vi "Translate to Array Data.vi"(0 "original data":path=path "C:/Users/User/Desktop/aaa.csv", 1 "Only Use Last Value?":bool=TRUE, 2 "Electrode number, N":u16=8, 3 "Current Mode":u8[][](array[numeric]), 5 "original error":errorcluster, 7 "Array Mode":u16(ring) items=["None", "Gradient + Dipole dipole", "Gradient", "Dipole Dipole", "Schlumberger"], 9 "modified data":path=path "C:/Users/User/Desktop/test.csv", 11 "modified error":errorcluster, 12 "Inverse\nPolarity":bool=TRUE, 13 "Insert\nBreak":bool=TRUE, 14 "External\nRef":bool=TRUE) -> ()   [LabVIEW 2023]
uses:
  <vilib>/Utility/error.llb/DialogType.ctl
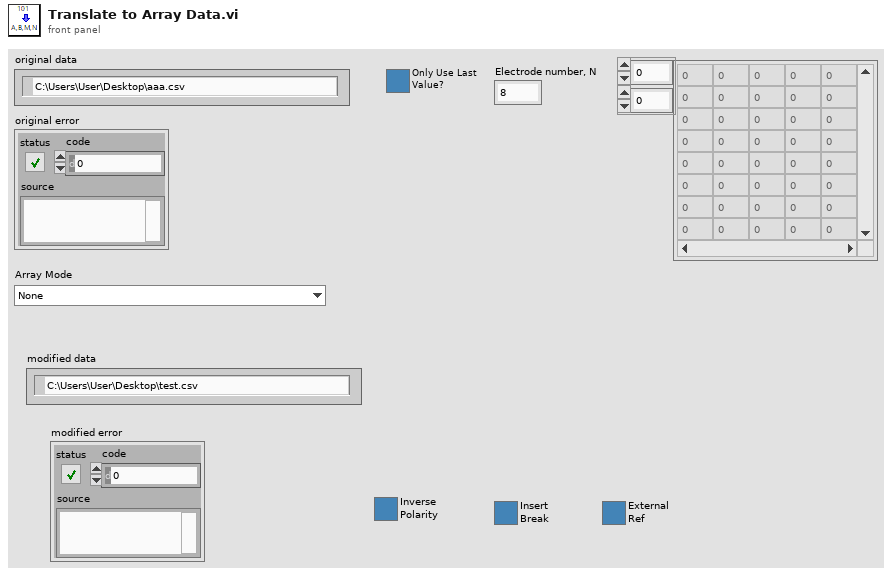
[diagram p1: front panel]
types:
  T1 = enum16{"open", "replace", "create", "open or create", "replace or create", "replace or create with confirmation"}
  T2 = typedef "DialogType.ctl" = u16
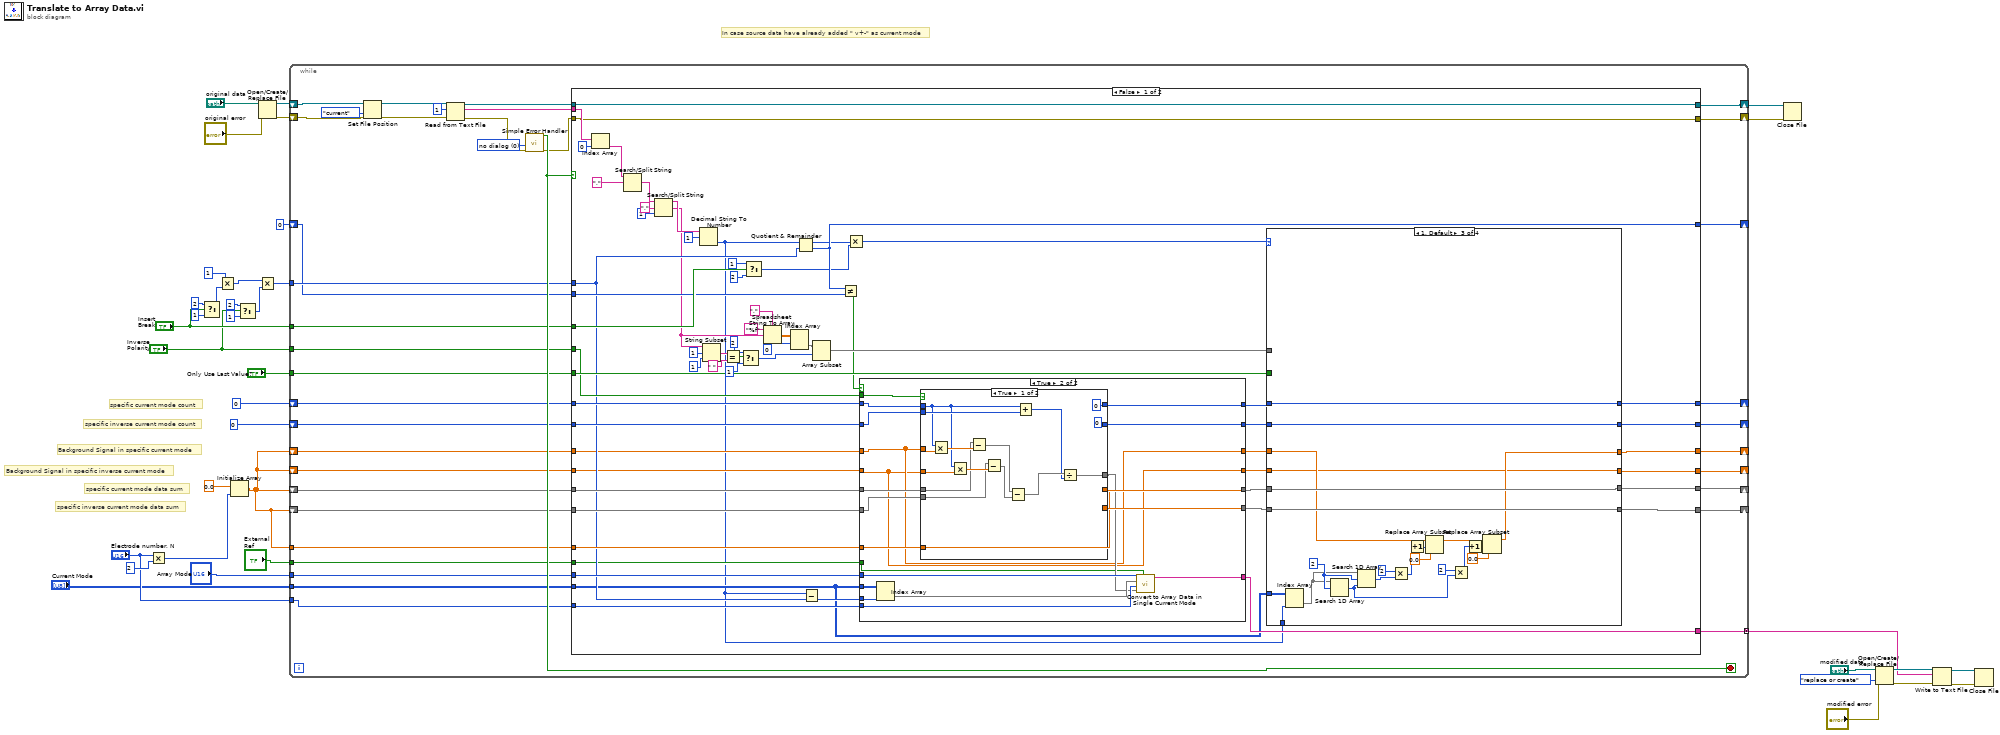
[diagram p0: block diagram]
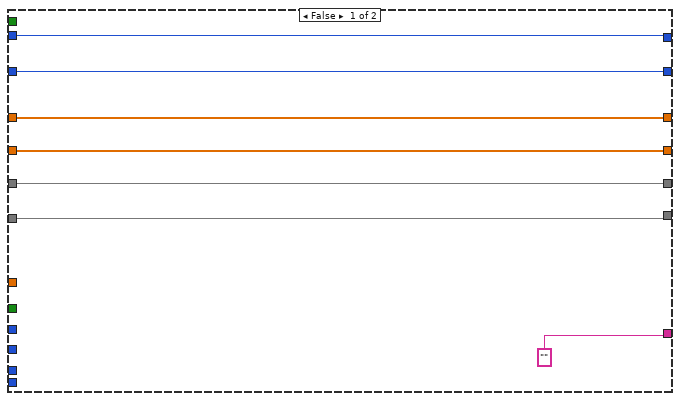
[diagram p2: hidden frame]
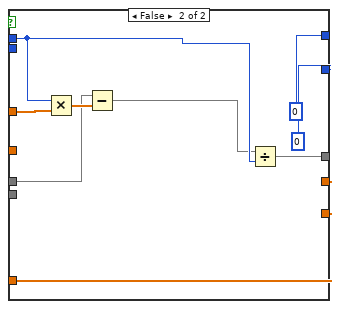
[diagram p3: hidden frame]
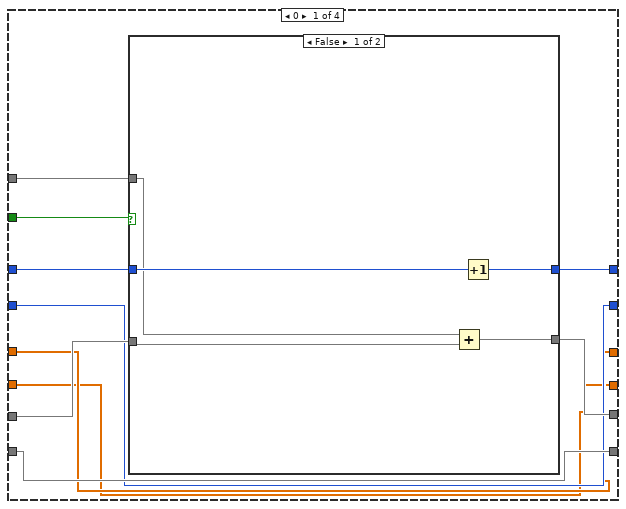
[diagram p4: hidden frame]
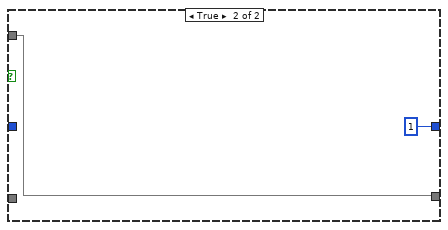
[diagram p5: hidden frame]
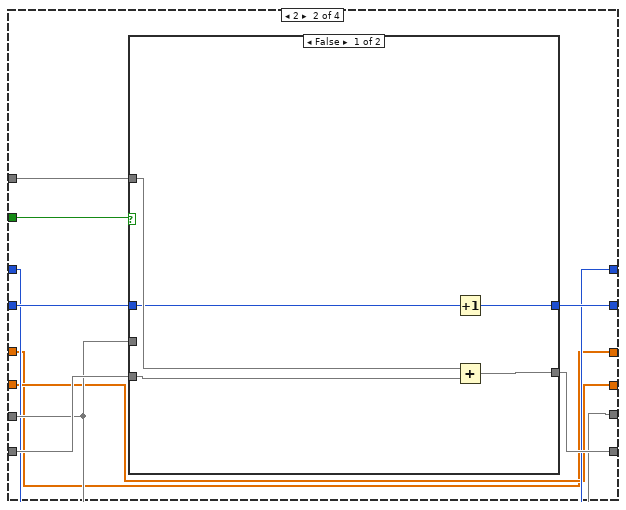
[diagram p6: hidden frame]
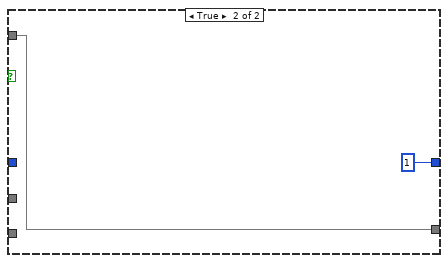
[diagram p7: hidden frame]
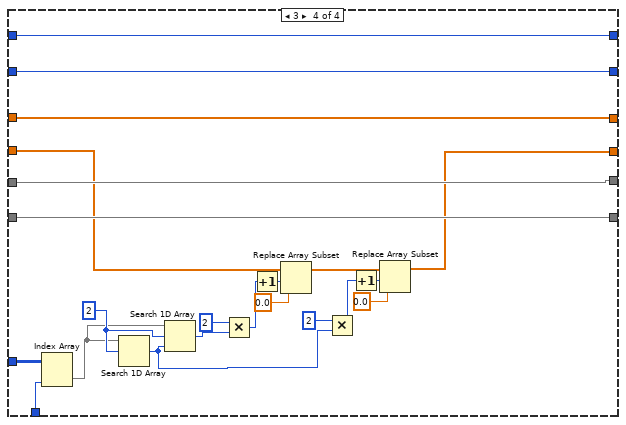
[diagram p8: hidden frame]
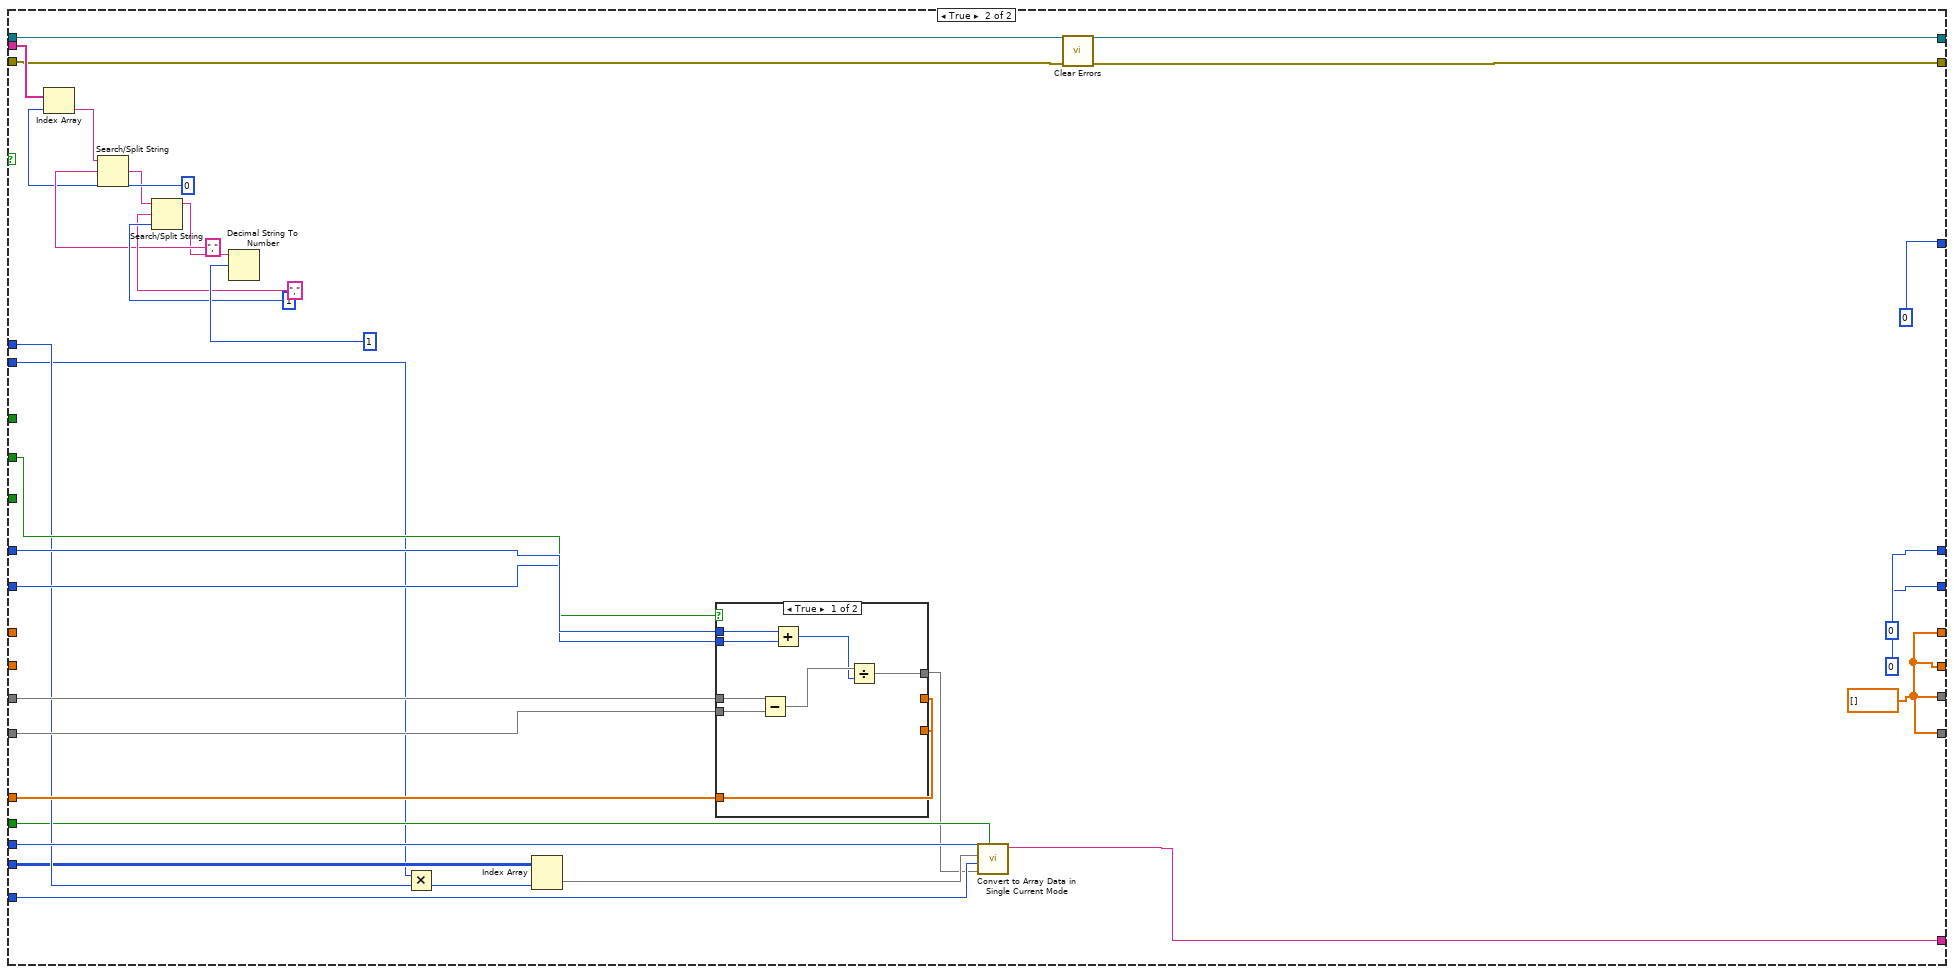
[diagram p9: hidden frame]
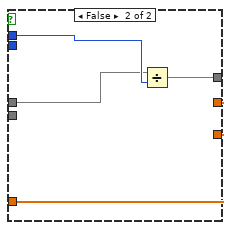
[diagram p10: hidden frame]
diagram:
  # "Background Signal in specific inverse current mode"
  # "Background Signal in specific current mode"
  # "In case source data have already added \" v+-\" as current mode"
  # "specific inverse current mode data sum"
  # "specific current mode data sum"
  # "specific inverse current mode count"
  # "specific current mode count"
  n1 = Multiply(x="Electrode number, N", y=u16 2) -> (x*y=w11:u16)
  n2 = Select(t=2 ("number"), s="Insert\nBreak", f=1 ("number")) -> (s? t:f=w20:i32)
  n3 = Multiply(x=1 ("number"), y=w20) -> (x*y=w14:i32)
  n4 = Initialize Array(0.0 ("element"), w11) -> (w1:dbl[])
  n5 = Select(t=2 ("number"), s="Inverse\nPolarity", f=1 ("number")) -> (s? t:f=w19:i32)
  n6 = Open/Create/Replace File(file path (use dialog)="original data", error in="original error") -> (refnum out=w34:refnum<file>, error out=w35:errorcluster)  [unwired: 4 in, 1 out]
  n7 = Multiply(x=w14, y=w19) -> (x*y=w18:i32)
  n8 = while {
    shift-right: [w67] -> w29
    shift-left: w35 -> [w74]
    shift-right: [w66] -> w36
    shift-left: w34 -> [w65]
    tunnel: "Insert\nBreak" -> [w61]
    tunnel: "Inverse\nPolarity" -> [w60]
    tunnel: "Only Use Last Value?" -> [w59]
    tunnel: w18 -> [w58]
    shift-right: [w53] -> _
    shift-left: 0 ("number") -> [w57]
    shift-right: [w50] -> _
    shift-left: 0 ("number") -> [w56]
    shift-right: [w52] -> _
    shift-left: w1 -> [w55]
    shift-right: [w51] -> _
    shift-left: w1 -> [w54]
    shift-right: [w49] -> _
    shift-left: 0 -> [w48]
    tunnel: w1 -> [w47]
    tunnel: "Current Mode" -> [w45]
    tunnel: "Array Mode" -> [w46]
    tunnel: "Electrode number, N" -> [w44]
    tunnel: "External\nRef" -> [w43]
    tunnel: [w42] -> w5 mode=concatenating
    shift-right: [w39] -> _
    shift-left: w1 -> [w41]
    shift-right: [w38] -> _
    shift-left: w1 -> [w40]
    stop <- w71 stop-if-true
    w72 = T2 0 items=["no dialog", "OK message", "continue or stop message", "OK message + warnings", "continue/stop + warnings"] ("type of dialog (OK msg:1)")
    n9 = Set File Position(refnum=w65, from (0:start)=enum16{"start", "end", "current"}."current", error in=w74) -> (refnum out=w64:refnum<file>, error out=w63:errorcluster)  [unwired: 1 in]
    n10 = Read from Text File(file (use dialog)=w64, count=1, error in=w63) -> (refnum out=w69:refnum<file>, text=w70:string[], error out=w68:errorcluster)  [unwired: 1 in, 1 out]
    n11 = call <vilib>:"Simple Error Handler.vi"("type of dialog (OK msg:1)"=w72, "error in (no error)"=w68) -> ("error?"=w71:bool, "error out"=w62:errorcluster)  [unwired: 3 in, 3 out]
    n12 = case shown="False" w71 {
      tunnel: w70 -> [w135 w297]
      tunnel: w69 -> [w132 w294]
      tunnel: w62 -> [w131 w276]
      tunnel: [w132 w294] -> w66
      tunnel: [w131 w275] -> w67
      tunnel: w61 -> [w128 _]
      tunnel: w60 -> [w108 w287]
      tunnel: w59 -> [w127 _]
      tunnel: w58 -> [w96 w283]
      tunnel: w57 -> [w112 w291]
      tunnel: w56 -> [w111 w290]
      tunnel: w55 -> [w110 w289]
      tunnel: w54 -> [w109 w288]
      tunnel: [w118 0 ("number")] -> w53
      tunnel: [w117 w270] -> w52
      tunnel: [w116 w270] -> w51
      tunnel: [w115 0 ("number")] -> w50
      tunnel: [w113 0] -> w49
      tunnel: w48 -> [w114 w271]
      tunnel: w47 -> [w102 w286]
      tunnel: w46 -> [w98 w285]
      tunnel: w45 -> [w79 w272]
      tunnel: w44 -> [w95 w282]
      tunnel: w43 -> [w94 w281]
      tunnel: [w93 w280] -> w42
      tunnel: w41 -> [w83 _]
      tunnel: w40 -> [w82 _]
      tunnel: [w77 w270] -> w39
      tunnel: [w76 w270] -> w38
      frame False {
        n13 = Index Array(array=w135, index=0) -> (element=w133:string)
        n14 = Search/Split String(string=w133, search string/char (-)=",") -> (match + rest of string=w123:string)  [unwired: 1 in, 2 out]
        n15 = Search/Split String(string=w123, search string/char (-)=",", offset (0)=1) -> (substring before match=w124:string, match + rest of string=w85:string)  [unwired: 1 out]
        n16 = Decimal String To Number(string=w124, offset=1) -> (number=w78:i32)  [unwired: 1 in, 1 out]
        n17 = String Subset(string=w85, offset (0)=1, length (rest)=1 ("length (rest)")) -> (substring=w92:string)
        n18 = Equal?(x=w92, y=" ") -> (x = y?=w91:bool)
        n19 = Select(t=2 ("index (row)"), s=w91, f=1 ("index (row)")) -> (s? t:f=w84:i32)
        n20 = Select(t=1, s=w128, f=2 ("y")) -> (s? t:f=w101:i32)
        n21 = Spreadsheet String To Array(delimiter (Tab)=",", format string="%f", spreadsheet string=w85) -> (array=w122:dbl[][])  [unwired: 1 in]
        n22 = Index Array(array=w122, index (row)=0) -> (element=w120:dbl[])  [unwired: 1 in]
        n23 = Quotient & Remainder(x=w78, y=w96) -> (x-y*floor(x/y)=w100:i32, floor(x/y)=w113:i32)
        n24 = Subtract(x=w78, y=w96) -> (x-y=w97:i32)
        n25 = Array Subset(array=w120, index=w84) -> (w119:dbl[])  [unwired: 1 in]
        n26 = Not Equal?(x=w113, y=w114) -> (x != y?=w103:bool)
        n27 = Multiply(x=w100, y=w101) -> (x*y=w99:i32)
        n28 = case shown="True" w103 {
          tunnel: w112 -> [w146 w163]
          tunnel: w111 -> [w145 w162]
          tunnel: w110 -> [w144 w165]
          tunnel: w109 -> [w143 w164]
          tunnel: w108 -> [_ w166]
          tunnel: [w146 w161] -> w107
          tunnel: [w145 w160] -> w106
          tunnel: [w144 w159] -> w105
          tunnel: [w143 w158] -> w104
          tunnel: w102 -> [_ w157]
          tunnel: w98 -> [_ w153]
          tunnel: w79 -> [_ w156]
          tunnel: w97 -> [_ w155]
          tunnel: w95 -> [_ w152]
          tunnel: w94 -> [_ w150]
          tunnel: ["" ("String") w149] -> w93
          tunnel: w83 -> [w141 w148]
          tunnel: w82 -> [w140 w147]
          tunnel: [w141 w148] -> w81
          tunnel: [w140 w147] -> w80
          frame False {
          }
          frame True {
            n29 = Index Array(array=w156, index (col)=w155) -> (element=w154:u8[])  [unwired: 1 in]
            n30 = case shown="True" w166 {
              tunnel: w165 -> [w170 w184]
              tunnel: w164 -> [w169 _]
              tunnel: w163 -> [w171 w186]
              tunnel: w162 -> [w182 _]
              tunnel: [0 ("number") 0 ("number")] -> w161
              tunnel: [0 ("number") 0 ("number")] -> w160
              tunnel: [w177 w189] -> w159
              tunnel: [w177 w189] -> w158
              tunnel: w157 -> [w177 w189]
              tunnel: [w176 w188] -> w151
              tunnel: w148 -> [w174 w187]
              tunnel: w147 -> [w172 _]
              frame True {
                n31 = Multiply(x=w171, y=w174) -> (x*y=w175:dbl[])
                n32 = Multiply(x=w171, y=w172) -> (x*y=w173:dbl[])
                n33 = Subtract(x=w170, y=w175) -> (x-y=w167:dbl[])
                n34 = Subtract(x=w169, y=w173) -> (x-y=w168:dbl[])
                n35 = Subtract(x=w167, y=w168) -> (x-y=w181:dbl[])
                n36 = Add(x=w171, y=w182) -> (x+y=w180:i32)
                n37 = Divide(x=w181, y=w180) -> (x/y=w176:dbl[])
              }
              frame False {
                n38 = Multiply(x=w186, y=w187) -> (x*y=w185:dbl[])
                n39 = Subtract(x=w184, y=w185) -> (x-y=w183:dbl[])
                n40 = Divide(x=w183, y=w186) -> (x/y=w188:dbl[])
              }
            }
            n41 = call "Convert to Array Data in Single Current Mode.vi"("External\nRef"=w150, "data"=w151, "Electrode number, N"=w152, "Current Mode"=w154, "Array Mode"=w153) -> ("String"=w149:string)  [unwired: 6 in]
          }
        }
        n42 = case shown="1, Default" w99 {
          tunnel: w127 -> [w201 w218 _ _]
          tunnel: w119 -> [w197 w217 _ _]
          tunnel: w107 -> [w200 w211 w247 w269]
          tunnel: w106 -> [w194 w214 w246 w268]
          tunnel: w105 -> [w199 w212 w245 w267]
          tunnel: w104 -> [w195 w216 w244 w266]
          tunnel: [w198 w211 w247 w269] -> w118
          tunnel: [w196 w212 w245 w267] -> w117
          tunnel: [w195 w215 w244 w266] -> w116
          tunnel: [w194 w213 w246 w268] -> w115
          tunnel: w81 -> [w193 w209 w239 w248]
          tunnel: w80 -> [w192 w210 w226 w250]
          tunnel: w79 -> [_ _ w241 w263]
          tunnel: w78 -> [_ _ w240 w262]
          tunnel: [w193 w209 w227 w248] -> w77
          tunnel: [w192 w210 w226 w249] -> w76
          frame 0 {
            n43 = case shown="False" w201 {
              tunnel: w200 -> [w206 _]
              tunnel: w199 -> [w203 _]
              tunnel: [w205 1 ("number")] -> w198
              tunnel: w197 -> [w202 w207]
              tunnel: [w204 w207] -> w196
              frame False {
                n44 = Add(x=w202, y=w203) -> (x+y=w204:dbl[])
                n45 = Increment(x=w206) -> (x+1=w205:i32)
              }
              frame True {
              }
            }
          }
          frame 2 {
            n46 = case shown="False" w218 {
              tunnel: w212 -> [_ _]
              tunnel: w217 -> [w222 w225]
              tunnel: [w223 w225] -> w215
              tunnel: w216 -> [w221 _]
              tunnel: w214 -> [w220 _]
              tunnel: [w219 1 ("number")] -> w213
              frame False {
                n47 = Increment(x=w220) -> (x+1=w219:i32)
                n48 = Add(x=w222, y=w221) -> (x+y=w223:dbl[])
              }
              frame True {
              }
            }
          }
          frame 1, Default {
            w243 = u8 2 ("element")
            n49 = Index Array(array=w241, index (col)=w240) -> (element=w242:u8[])  [unwired: 1 in]
            n50 = Search 1D Array(1D array=w242, element=w243) -> (index of element=w228:i32)  [unwired: 1 in]
            n51 = Search 1D Array(1D array=w242, element=w243, start index (0)=w228) -> (index of element=w238:i32)
            n52 = Multiply(x=2, y=w238) -> (x*y=w236:i32)
            n53 = Increment(x=w236) -> (x+1=w235:i32)
            n54 = Replace Array Subset(array=w239, new element=0.0 ("new element/subarray"), index=w235) -> (w231:dbl[])
            n55 = Multiply(x=2, y=w228) -> (x*y=w229:i32)
            n56 = Increment(x=w229) -> (x+1=w232:i32)
            n57 = Replace Array Subset(array=w231, new element=0.0 ("new element/subarray"), index=w232) -> (w227:dbl[])
          }
          frame 3 {
            w265 = u8 2 ("element")
            n58 = Index Array(array=w263, index (col)=w262) -> (element=w264:u8[])  [unwired: 1 in]
            n59 = Search 1D Array(1D array=w264, element=w265) -> (index of element=w251:i32)  [unwired: 1 in]
            n60 = Search 1D Array(1D array=w264, element=w265, start index (0)=w251) -> (index of element=w261:i32)
            n61 = Multiply(x=2, y=w261) -> (x*y=w259:i32)
            n62 = Increment(x=w259) -> (x+1=w258:i32)
            n63 = Replace Array Subset(array=w250, new element=0.0 ("new element/subarray"), index=w258) -> (w254:dbl[])
            n64 = Multiply(x=2, y=w251) -> (x*y=w252:i32)
            n65 = Increment(x=w252) -> (x+1=w255:i32)
            n66 = Replace Array Subset(array=w254, new element=0.0 ("new element/subarray"), index=w255) -> (w249:dbl[])
          }
        }
      }
      frame True {
        w270 = dbl[] [] ("subarray")
        n67 = Index Array(array=w297, index=0) -> (element=w295:string)
        n68 = Search/Split String(string=w295, search string/char (-)=",") -> (match + rest of string=w292:string)  [unwired: 1 in, 2 out]
        n69 = Search/Split String(string=w292, search string/char (-)=",", offset (0)=1) -> (substring before match=w293:string)  [unwired: 2 out]
        n70 = Decimal String To Number(string=w293, offset=1) -> ()  [unwired: 1 in, 2 out]
        n71 = Multiply(x=w271, y=w283) -> (x*y=w284:i32)
        n72 = Index Array(array=w272, index (col)=w284) -> (element=w274:u8[])  [unwired: 1 in]
        n73 = case shown="True" w287 {
          tunnel: w289 -> [w309 w312]
          tunnel: w288 -> [w308 _]
          tunnel: w291 -> [w307 w313]
          tunnel: w290 -> [w306 _]
          tunnel: [w303 w311] -> _
          tunnel: [w303 w311] -> _
          tunnel: w286 -> [w303 w311]
          tunnel: [w302 w310] -> w273
          frame True {
            n74 = Subtract(x=w309, y=w308) -> (x-y=w305:dbl[])
            n75 = Add(x=w307, y=w306) -> (x+y=w304:i32)
            n76 = Divide(x=w305, y=w304) -> (x/y=w302:dbl[])
          }
          frame False {
            n77 = Divide(x=w312, y=w313) -> (x/y=w310:dbl[])
          }
        }
        n78 = call "Convert to Array Data in Single Current Mode.vi"("External\nRef"=w281, "data"=w273, "Electrode number, N"=w282, "Current Mode"=w274, "Array Mode"=w285) -> ("String"=w280:string)  [unwired: 6 in]
        n79 = call <vilib>:"Clear Errors.vi"("error in (no error)"=w276) -> ("error out"=w275:errorcluster)  [unwired: 5 in, 1 out]
      }
    }
  }
  n80 = Close File(refnum=w36, error in=w29) -> ()  [unwired: 2 out]
  n81 = Open/Create/Replace File(file path (use dialog)="modified data", error in="modified error", operation (0:open)=T1."replace or create") -> (refnum out=w7:refnum<file>, error out=w6:errorcluster)  [unwired: 3 in, 1 out]
  n82 = Write to Text File(file (use dialog)=w7, text=w5, error in=w6) -> (refnum out=w4:refnum<file>, error out=w3:errorcluster)  [unwired: 1 in, 1 out]
  n83 = Close File(refnum=w4, error in=w3) -> ()  [unwired: 2 out]
